vi "Teleop.vi"(10 "Match Info":T1={"Autonomous Elapsed Seconds"=0.0, "TeleOp Elapsed Seconds"=0.0, "Disabled Elapsed Seconds"=0.0, "Visited Autonomous"=FALSE, "Visited TeleOp"=FALSE, "Visited Disabled"=FALSE, "Autonomous Settings"={"Autonomous Style"=enum."Independent", "VI Refnum"=refnum}}, 11 "Call Context":T2) -> ()   [LabVIEW 2011]
doc: "This VI is called for each TeleOp packet received from the DS where the robot is not disabled. It is often used to read from the joysticks and update I/O or to update setpoints for timed control loops. It should complete and return within 20 milliseconds or it may miss DS packets."
uses:
  <vilib>/Rock Robotics/WPI/DriverStation/WPI_DriverStationDerivedRobotMode.ctl
  <vilib>/Rock Robotics/WPI/DriverStation/WPI_DriverStationMatch Info.ctl
  Robot Global Data.vi
panel:
  in  "x":dbl=0.25
  out "Position 4":dbl
  out "Position 3":dbl
  out "Shift Control":dbl=2.0 format="%.2f"
  in  "Left High":dbl=0.2
  in  "Right High":dbl=0.8
  in  "Left Mid":dbl=0.25
  in  "Right Mid":dbl=0.7
  in  "Shift Input 2":dbl
  in  "Left Low":dbl=0.8
  in  "Right Low":dbl=0.4
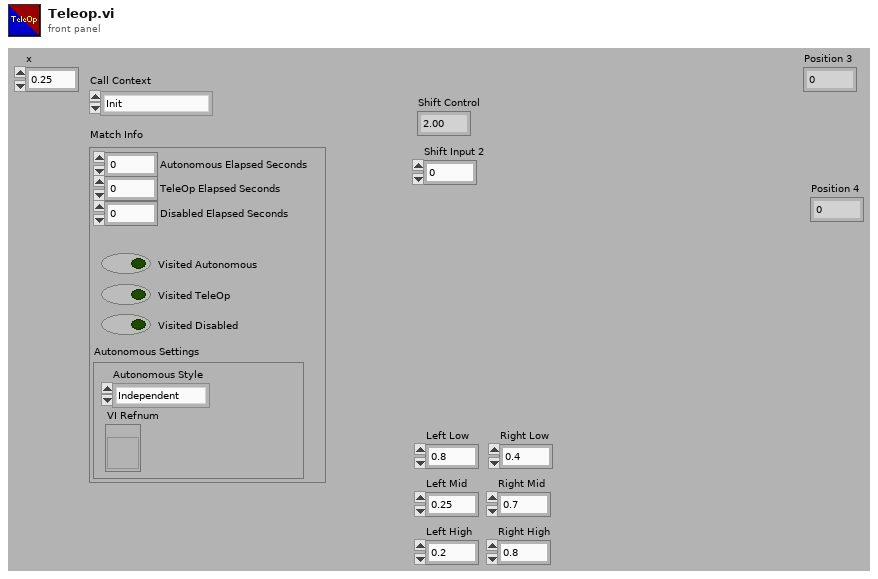
[diagram p1: front panel]
types:
  T1 = typedef "WPI_DriverStationMatch Info.ctl" = cluster{"Autonomous Elapsed Seconds":dbl, "TeleOp Elapsed Seconds":dbl, "Disabled Elapsed Seconds":dbl, "Visited Autonomous":bool, "Visited TeleOp":bool, "Visited Disabled":bool, "Autonomous Settings":cluster{"Autonomous Style":enum16{"Iterative", "Independent"}, "VI Refnum":refnum<vi>}}
  T2 = typedef "WPI_DriverStationDerivedRobotMode.ctl" = enum16{"Init", "Execute", "Stop"}
  T3 = typedef "WPI_MotorControlDeviceRef.ctl" = cluster{"DeviceStatus":errorcluster, "Type":enum16{"PWM", "CAN"}, "PWM":cluster{"Digital Module":T4, "PWM Channel":T5, "DeadBand":T6}, "CAN":cluster{"Device Number":u8, "Control Mode":T7, "Semaphore":T8, "Max Vout":dbl}, "Invert":bool, "TransformRef":T9, "InvTransformRef":T9}
  T4 = typedef "FPGA_TypedefDigitalModule.ctl" = enum16{"Digital Module 1", "Digital Module 2"}
  T5 = typedef "FPGA_DIOPWMChannel.ctl" = enum8{"PWM 1", "PWM 2", "PWM 3", "PWM 4", "PWM 5", "PWM 6", "PWM 7", "PWM 8", "PWM 9", "PWM 10", "Invalid"}
  T6 = typedef "WPI_PWMDeadband.ctl" = cluster{"Name":string, "maxPositivePwm":i32, "minPositivePwm":i32, "centerPwm":i32, "maxNegativePwm":i32, "minNegativePwm":i32, "angularRange":u16}
  T7 = typedef "WPI_CANJaguar_ControlMode.ctl" = enum8{"Percent VBus", "Current", "Speed", "Position", "Voltage"}
  T8 = typedef "Semaphore RefNum" = refnum<k1>
  T9 = typedef "WPI_PWMTransform_ConPane.ctl" = refnum<vi>
  T10 = typedef "WPI_JoystickDevRef.ctl" = cluster{"Device":T11}
  T11 = typedef "WPI_JoystickDeviceEnum.ctl" = enum16{"USB 1", "USB 2", "USB 3", "USB 4", "Kinect 1", "Kinect 2"}
  T12 = typedef "WPI_JoystickButtonState.ctl" = cluster{"Button 1":bool, "Button 2":bool, "Button 3":bool, "Button 4":bool, "Button 5":bool, "Button 6":bool, "Button 7":bool, "Button 8":bool, "Button 9":bool, "Button 10":bool, "Button 11":bool, "Button 12":bool}
  T13 = cluster{"axis 1 (x)":dbl, "axis 2 (y)":dbl, "axis 3 (throttle)":dbl, "axis 4":dbl, "axis 5":dbl, "axis 6":dbl}
  T14 = typedef "WPI_DigitalInputDevRef.ctl" = cluster{"DevStatus":errorcluster, "DIO Channel":T15, "Digital Module":T4}
  T15 = typedef "FPGA_DIOChannel.ctl" = enum8{"DIO 1", "DIO 2", "DIO 3", "DIO 4", "DIO 5", "DIO 6", "DIO 7", "DIO 8", "DIO 9", "DIO 10", "DIO 11", "DIO 12", "DIO 13", "DIO 14", "Invalid"}
  T16 = typedef "WPI_ServoDeviceRef.ctl" = cluster{"DeviceStatus":errorcluster, "Digital Module":T4, "PWM Channel":T5, "DeadBand":T6}
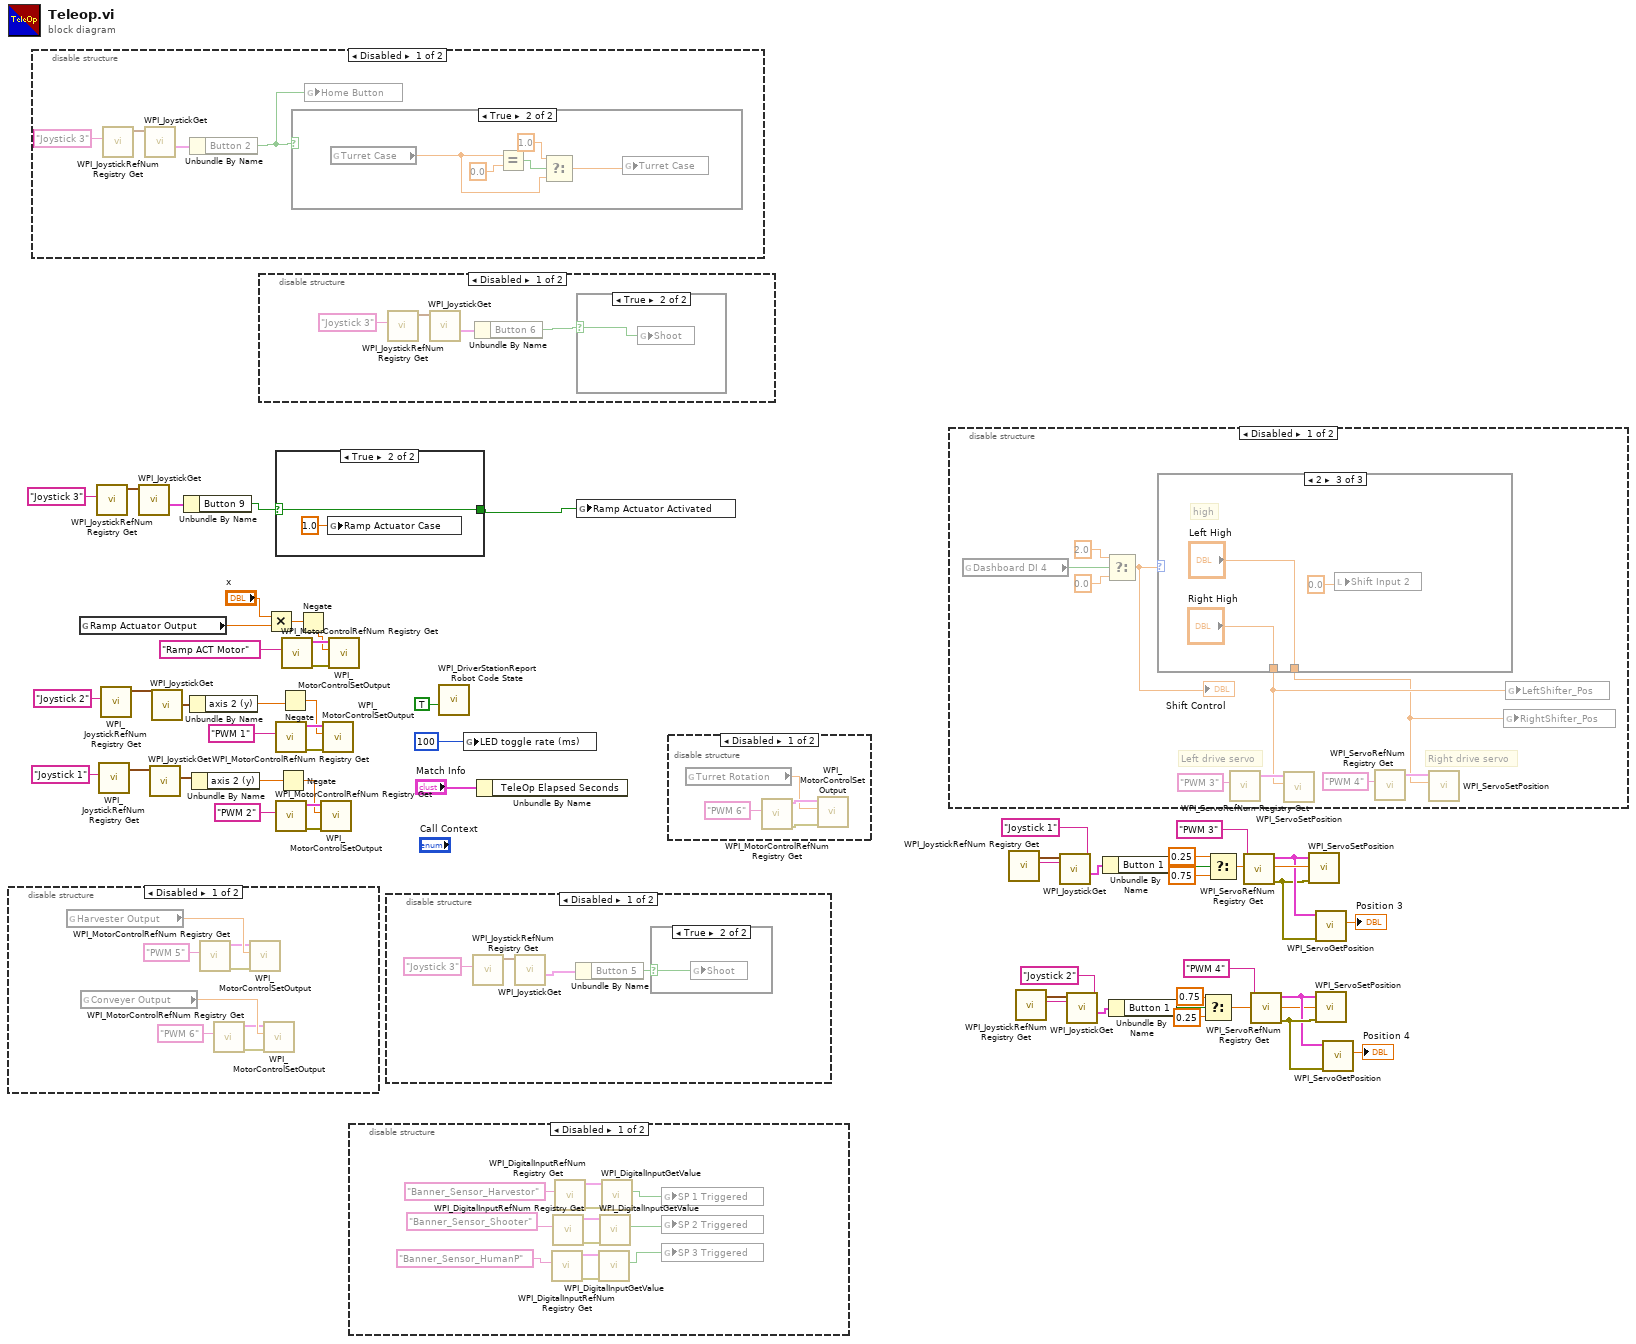
[diagram p0: block diagram]
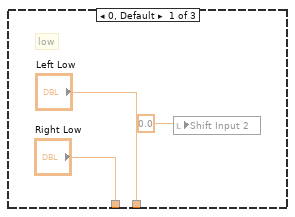
[diagram p12: hidden frame]
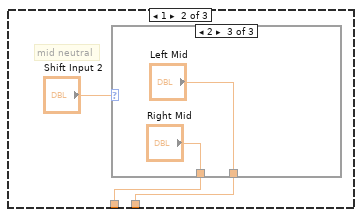
[diagram p13: hidden frame]
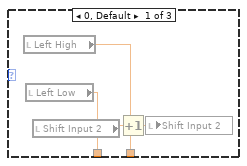
[diagram p14: hidden frame]
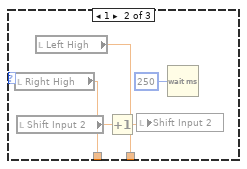
[diagram p15: hidden frame]
diagram:
  n1 = disable-structure shown="Disabled" {
    frame Disabled {
      n2 = global read "Robot Global Data.vi" "Harvester Output"() -> (w59:dbl)
      n3 = global read "Robot Global Data.vi" "Conveyer Output"() -> (w55:dbl)
      n4 = call <vilib>:"WPI_MotorControlRefNum Registry Get.vi"("refnum name"="PWM 5") -> ("error out"=w60:errorcluster, "MotorControlDevRef"=w58:T3)  [unwired: 9 in]
      n5 = call <vilib>:"WPI_MotorControlRefNum Registry Get.vi"("refnum name"="PWM 6") -> ("error out"=w56:errorcluster, "MotorControlDevRef"=w54:T3)  [unwired: 9 in]
      n6 = call <vilib>:"WPI_MotorControlSetOutput.vi"("error in (no error)"=w60, "Output"=w59, "MotorControlDevRef"=w58) -> ()  [unwired: 7 in, 2 out]
      n7 = call <vilib>:"WPI_MotorControlSetOutput.vi"("error in (no error)"=w56, "Output"=w55, "MotorControlDevRef"=w54) -> ()  [unwired: 7 in, 2 out]
    }
    frame Enabled {
    }
  }
  n8 = disable-structure shown="Disabled" {
    frame Disabled {
      n9 = call <vilib>:"WPI_JoystickRefNum Registry Get.vi"("refnum name"="Joystick 3") -> ("JoystickDevRef"=w63:T10)  [unwired: 9 in, 1 out]
      n10 = call <vilib>:"WPI_JoystickGet.vi"("JoystickDevRef"=w63) -> ("Buttons"=w64:T12)  [unwired: 4 in, 2 out]
      n11 = Unbundle By Name(w64) -> ("Button 2"=w62:bool)
      n12 = case shown="True" w62 {
        frame False {
        }
        frame True {
          n13 = global read "Robot Global Data.vi" "Turret Case"() -> (w67:dbl)
          n14 = Equal?(x=w67, y=0.0) -> (x = y?=w69:bool)
          n15 = Select(t=1.0, s=w69, f=w67) -> (s? t:f=w66:dbl)
          n16 = global write "Robot Global Data.vi" "Turret Case"(w66) -> ()
        }
      }
      n17 = global write "Robot Global Data.vi" "Home Button"(w62) -> ()
    }
    frame Enabled {
    }
  }
  n18 = global read "Robot Global Data.vi" "Ramp Actuator Output"() -> (w7:dbl)
  n19 = call <vilib>:"WPI_JoystickRefNum Registry Get.vi"("refnum name"="Joystick 3") -> ("JoystickDevRef"=w12:T10)  [unwired: 9 in, 1 out]
  n20 = call <vilib>:"WPI_JoystickRefNum Registry Get.vi"("refnum name"="Joystick 1") -> ("JoystickDevRef"=w45:T10)  [unwired: 9 in, 1 out]
  n21 = call <vilib>:"WPI_JoystickRefNum Registry Get.vi"("refnum name"="Joystick 2") -> ("JoystickDevRef"=w48:T10)  [unwired: 9 in, 1 out]
  n22 = call <vilib>:"WPI_JoystickGet.vi"("JoystickDevRef"=w12) -> ("Buttons"=w11:T12)  [unwired: 4 in, 2 out]
  n23 = call <vilib>:"WPI_JoystickGet.vi"("JoystickDevRef"=w45) -> ("Axes"=w49:T13)  [unwired: 4 in, 2 out]
  n24 = call <vilib>:"WPI_JoystickGet.vi"("JoystickDevRef"=w48) -> ("Axes"=w50:T13)  [unwired: 4 in, 2 out]
  n25 = Unbundle By Name(w11) -> ("Button 9"=w2:bool)
  n26 = Unbundle By Name(w50) -> ("axis 2 (y)"=w38:dbl)
  n27 = Unbundle By Name(w49) -> ("axis 2 (y)"=w36:dbl)
  n28 = disable-structure shown="Disabled" {
    frame Disabled {
      n29 = call <vilib>:"WPI_JoystickRefNum Registry Get.vi"("refnum name"="Joystick 3") -> ("JoystickDevRef"=w73:T10)  [unwired: 9 in, 1 out]
      n30 = call <vilib>:"WPI_JoystickGet.vi"("JoystickDevRef"=w73) -> ("Buttons"=w72:T12)  [unwired: 4 in, 2 out]
      n31 = Unbundle By Name(w72) -> ("Button 6"=w74:bool)
      n32 = case shown="True" w74 {
        selector: w74 -> [_ w75]
        frame False {
        }
        frame True {
          n33 = global write "Robot Global Data.vi" "Shoot"(w75) -> ()
        }
      }
    }
    frame Enabled {
    }
  }
  n34 = Multiply(x="x", y=w7) -> (x*y=w4:dbl)
  n35 = case shown="True" w2 {
    selector: w2 -> [w76 w78]
    tunnel: [w76 w78] -> w1
    frame False {
    }
    frame True {
      n36 = global write "Robot Global Data.vi" "Ramp Actuator Case"(1.0 ("Ramp Actuator Case")) -> ()
    }
  }
  n37 = call <vilib>:"WPI_MotorControlRefNum Registry Get.vi"("refnum name"="PWM 1") -> ("error out"=w42:errorcluster, "MotorControlDevRef"=w41:T3)  [unwired: 9 in]
  n38 = call <vilib>:"WPI_MotorControlRefNum Registry Get.vi"("refnum name"="PWM 2") -> ("error out"=w44:errorcluster, "MotorControlDevRef"=w43:T3)  [unwired: 9 in]
  n39 = Negate(x=w36) -> (-x=w35:dbl)
  n40 = Negate(x=w38) -> (-x=w37:dbl)
  n41 = call <vilib>:"WPI_MotorControlRefNum Registry Get.vi"("refnum name"="Ramp ACT Motor") -> ("error out"=w8:errorcluster, "MotorControlDevRef"=w5:T3)  [unwired: 9 in]
  n42 = Negate(x=w4) -> (-x=w3:dbl)
  n43 = call <vilib>:"WPI_MotorControlSetOutput.vi"("error in (no error)"=w44, "Output"=w35, "MotorControlDevRef"=w43) -> ()  [unwired: 7 in, 2 out]
  n44 = call <vilib>:"WPI_MotorControlSetOutput.vi"("error in (no error)"=w42, "Output"=w37, "MotorControlDevRef"=w41) -> ()  [unwired: 7 in, 2 out]
  n45 = call <vilib>:"WPI_MotorControlSetOutput.vi"("error in (no error)"=w8, "Output"=w3, "MotorControlDevRef"=w5) -> ()  [unwired: 7 in, 2 out]
  n46 = disable-structure shown="Disabled" {
    frame Disabled {
      n47 = call <vilib>:"WPI_DigitalInputRefNum Registry Get.vi"("refnum name"="Banner_Sensor_HumanP") -> ("error out"=w85:errorcluster, "DigitalInputDevRef"=w84:T14)  [unwired: 9 in]
      n48 = call <vilib>:"WPI_DigitalInputRefNum Registry Get.vi"("refnum name"="Banner_Sensor_Shooter") -> ("error out"=w86:errorcluster, "DigitalInputDevRef"=w87:T14)  [unwired: 9 in]
      n49 = call <vilib>:"WPI_DigitalInputRefNum Registry Get.vi"("refnum name"="Banner_Sensor_Harvestor") -> ("error out"=w90:errorcluster, "DigitalInputDevRef"=w89:T14)  [unwired: 9 in]
      n50 = call <vilib>:"WPI_DigitalInputGetValue.vi"("error in (no error)"=w85, "DigitalInputDevRef"=w84) -> ("Value"=w82:bool)  [unwired: 7 in, 2 out]
      n51 = call <vilib>:"WPI_DigitalInputGetValue.vi"("error in (no error)"=w86, "DigitalInputDevRef"=w87) -> ("Value"=w83:bool)  [unwired: 7 in, 2 out]
      n52 = call <vilib>:"WPI_DigitalInputGetValue.vi"("error in (no error)"=w90, "DigitalInputDevRef"=w89) -> ("Value"=w88:bool)  [unwired: 7 in, 2 out]
      n53 = global write "Robot Global Data.vi" "SP 1 Triggered"(w88) -> ()
      n54 = global write "Robot Global Data.vi" "SP 2 Triggered"(w83) -> ()
      n55 = global write "Robot Global Data.vi" "SP 3 Triggered"(w82) -> ()
    }
    frame Enabled {
    }
  }
  n56 = disable-structure shown="Disabled" {
    frame Disabled {
      n57 = call <vilib>:"WPI_JoystickRefNum Registry Get.vi"("refnum name"="Joystick 3") -> ("JoystickDevRef"=w92:T10)  [unwired: 9 in, 1 out]
      n58 = call <vilib>:"WPI_JoystickGet.vi"("JoystickDevRef"=w92) -> ("Buttons"=w93:T12)  [unwired: 4 in, 2 out]
      n59 = Unbundle By Name(w93) -> ("Button 5"=w91:bool)
      n60 = case shown="True" w91 {
        selector: w91 -> [_ w95]
        frame False {
        }
        frame True {
          n61 = global write "Robot Global Data.vi" "Shoot"(w95) -> ()
        }
      }
    }
    frame Enabled {
    }
  }
  n62 = call <vilib>:"WPI_DriverStationReport Robot Code State.vi"("TeleOp"=TRUE ("Autonomous")) -> ()  [unwired: 10 in, 1 out]
  n63 = global write "Robot Global Data.vi" "LED toggle rate (ms)"(u32 100 ("LED ms toggle rate")) -> ()
  n64 = Unbundle By Name("Match Info") -> ()  [unwired: 1 out]
  n65 = global write "Robot Global Data.vi" "Ramp Actuator Activated"(w1) -> ()
  n66 = disable-structure shown="Disabled" {
    frame Disabled {
      n67 = global read "Robot Global Data.vi" "Turret Rotation"() -> (w96:dbl)
      n68 = call <vilib>:"WPI_MotorControlRefNum Registry Get.vi"("refnum name"="PWM 6") -> ("error out"=w99:errorcluster, "MotorControlDevRef"=w98:T3)  [unwired: 9 in]
      n69 = call <vilib>:"WPI_MotorControlSetOutput.vi"("error in (no error)"=w99, "Output"=w96, "MotorControlDevRef"=w98) -> ()  [unwired: 7 in, 2 out]
    }
    frame Enabled {
    }
  }
  n70 = disable-structure shown="Disabled" {
    frame Disabled {
      # "Right drive servo"
      # "Left drive servo"
      n71 = global read "Robot Global Data.vi" "Dashboard DI 4"() -> (w102:bool)
      n72 = Select(t=2.0, s=w102, f=0.0) -> (s? t:f=w104:dbl)
      "Shift Control" <- w104
      n73 = case shown="2" w104 {
        tunnel: ["Left Low" w114 "Left High"] -> w100
        tunnel: ["Right Low" w113 "Right High"] -> w101
        frame 0, Default {
          # "low"
          n74 = local write "Shift Input 2"(0.0 ("Input 2")) -> ()
        }
        frame 1 {
          # "mid neutral"
          n75 = case shown="2" "Shift Input 2" {
            tunnel: [w119 w120 "Left Mid"] -> w114
            tunnel: [w118 w121 "Right Mid"] -> w113
            frame 0, Default {
              n76 = local read "Left High"() -> (w119:dbl)
              n77 = local read "Left Low"() -> (w118:dbl)
              n78 = local read "Shift Input 2"() -> (w117:dbl)
              n79 = Increment(x=w117) -> (x+1=w116:dbl)
              n80 = local write "Shift Input 2"(w116) -> ()
            }
            frame 1 {
              n81 = local read "Right High"() -> (w121:dbl)
              n82 = local read "Shift Input 2"() -> (w123:dbl)
              n83 = local read "Left High"() -> (w120:dbl)
              n84 = Increment(x=w123) -> (x+1=w122:dbl)
              n85 = local write "Shift Input 2"(w122) -> ()
              n86 = Wait (ms)(milliseconds to wait=u32 250) -> ()  [unwired: 1 out]
            }
            frame 2 {
            }
          }
        }
        frame 2 {
          # "high"
          n87 = local write "Shift Input 2"(0.0 ("Input 2")) -> ()
        }
      }
      n88 = call <vilib>:"WPI_ServoRefNum Registry Get.vi"("refnum name"="PWM 3") -> ("ServoDeviceRef"=w109:T16)  [unwired: 1 in, 9 out]
      n89 = call <vilib>:"WPI_ServoSetPosition.vi"("Position"=w101, "ServoDeviceRef"=w109) -> ()  [unwired: 1 in, 9 out]
      n90 = call <vilib>:"WPI_ServoRefNum Registry Get.vi"("refnum name"="PWM 4") -> ("ServoDeviceRef"=w105:T16)  [unwired: 1 in, 9 out]
      n91 = call <vilib>:"WPI_ServoSetPosition.vi"("Position"=w100, "ServoDeviceRef"=w105) -> ()  [unwired: 1 in, 9 out]
      n92 = global write "Robot Global Data.vi" "RightShifter_Pos"(w100) -> ()
      n93 = global write "Robot Global Data.vi" "LeftShifter_Pos"(w101) -> ()
    }
    frame Enabled {
    }
  }
  n94 = call <vilib>:"WPI_JoystickRefNum Registry Get.vi"("refnum name"="Joystick 1") -> ("JoystickDevRef"=w34:T10)  [unwired: 9 in, 1 out]
  n95 = call <vilib>:"WPI_JoystickRefNum Registry Get.vi"("refnum name"="Joystick 2") -> ("JoystickDevRef"=w13:T10)  [unwired: 9 in, 1 out]
  n96 = call <vilib>:"WPI_JoystickGet.vi"("JoystickDevRef"=w34) -> ("Buttons"=w32:T12)  [unwired: 4 in, 2 out]
  n97 = call <vilib>:"WPI_JoystickGet.vi"("JoystickDevRef"=w13) -> ("Buttons"=w15:T12)  [unwired: 4 in, 2 out]
  n98 = Unbundle By Name(w32) -> ("Button 1"=w31:bool)
  n99 = Unbundle By Name(w15) -> ("Button 1"=w16:bool)
  n100 = Select(t=0.75, s=w16, f=0.25) -> (s? t:f=w19:dbl)
  n101 = Select(t=0.25, s=w31, f=0.75) -> (s? t:f=w28:dbl)
  n102 = call <vilib>:"WPI_ServoRefNum Registry Get.vi"("refnum name"="PWM 3") -> ("error out"=w25:errorcluster, "ServoDeviceRef"=w26:T16)  [unwired: 9 in]
  n103 = call <vilib>:"WPI_ServoRefNum Registry Get.vi"("refnum name"="PWM 4") -> ("error out"=w22:errorcluster, "ServoDeviceRef"=w21:T16)  [unwired: 9 in]
  n104 = call <vilib>:"WPI_ServoSetPosition.vi"("error in (no error)"=w25, "Position"=w28, "ServoDeviceRef"=w26) -> ()  [unwired: 7 in, 2 out]
  n105 = call <vilib>:"WPI_ServoGetPosition.vi"("error in (no error)"=w25, "ServoDeviceRef"=w26) -> ("Position"=→"Position 3":dbl)  [unwired: 7 in, 2 out]
  n106 = call <vilib>:"WPI_ServoSetPosition.vi"("error in (no error)"=w22, "Position"=w19, "ServoDeviceRef"=w21) -> ()  [unwired: 7 in, 2 out]
  n107 = call <vilib>:"WPI_ServoGetPosition.vi"("error in (no error)"=w22, "ServoDeviceRef"=w21) -> ("Position"=→"Position 4":dbl)  [unwired: 7 in, 2 out]
